vi "PCsName.vi"() -> (0 "Computer Name":string)   [LabVIEW 2015]
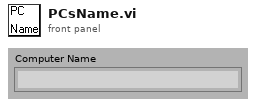
[diagram p1: front panel]
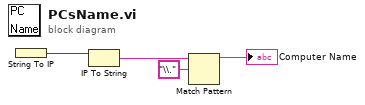
[diagram p0: block diagram]
diagram:
  n1 = String To IP() -> (0:w4:u32)  [unwired: 1 in]
  n2 = IP To String(2:w4) -> (0:w3:string)  [unwired: 1 in]
  n3 = Match Pattern(string=w3, regular expression="\\.") -> (before substring=→"Computer Name":string)  [unwired: 1 in, 3 out]
